vi "getPointFromEnemyOrientationAndBallToOurGoal.vi"(8 "error in (no error)":errorcluster, 9 "Robot":refnum<class "Robot.lvclass">, 10 "Game":refnum<class "Game.lvclass">, 11 "Utilities in":refnum<class "Utilities.lvclass">) -> (0 "error out":errorcluster, 1 "y_intersection":dbl, 2 "x_intersection":dbl, 3 "Utilities out":refnum<class "Utilities.lvclass">)   [LabVIEW 2018, in "Utilities.lvclass"]
uses:
  Utilities.lvclass
  Game_class/Game.lvclass
  Robot_class/Robot.lvclass
  Game_class/Game.lvclass/Game.ctl
  Robot_class/Robot.lvclass/Robot.ctl
  Object_class/Object.lvclass/Object.ctl
  Robot_class/Read orientation.vi
  Game_class/Read FieldRef.vi
  Game_class/Read BallRef.vi
  Object_class/Read x.vi
  Object_class/Read y.vi
  Ball_class/Ball.lvclass
  C:/Users/Gustavo/Desktop/RoboIME/SimplePass/SSL_AI/Object_class/Object.lvclass
  Field_class/Field.lvclass
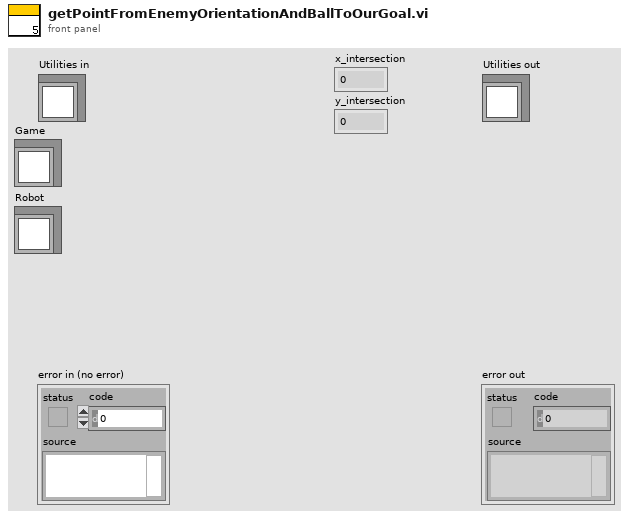
[diagram p1: front panel]
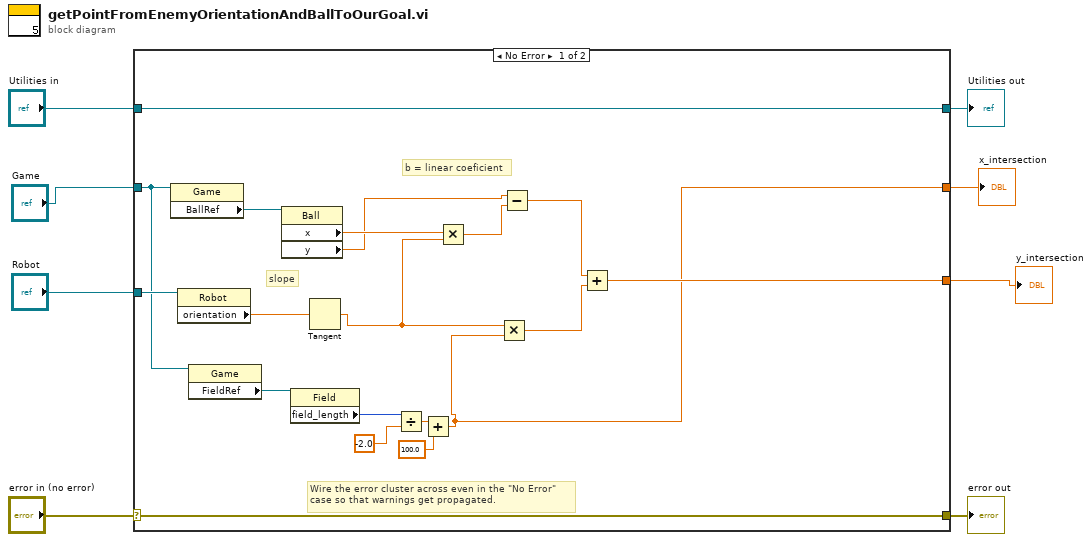
[diagram p0: block diagram]
diagram:
  n1 = case shown="No Error" "error in (no error)" {
    selector: "error in (no error)" -> [w26 w29]
    tunnel: [w26 w29] -> w7
    tunnel: [w27 w28] -> w5
    tunnel: "Utilities in" -> [w27 w28]
    tunnel: "Game" -> [w22 _]
    tunnel: "Robot" -> [w24 _]
    tunnel: [w11 _] -> w2
    tunnel: [w12 _] -> w1
    frame No Error {
      # "slope"
      # "b = linear coeficient"
      # "Wire the error cluster across even in the \"No Error\"\ncase so that warnings get propagated."
      n2 = property class="Game"(reference=w22) -> ("BallRef"=w25:refnum<class "Ball.lvclass">)  [unwired: 1 in, 2 out]
      n3 = property class="Robot"(reference=w24) -> ("orientation"=w23:dbl)  [unwired: 1 in, 2 out]
      n4 = property class="Game"(reference=w22) -> ("FieldRef"=w21:refnum<class "Field.lvclass">)  [unwired: 1 in, 2 out]
      n5 = property class="Ball"(reference=w25) -> ("x"=w18:dbl, "y"=w16:dbl)  [unwired: 1 in, 2 out]
      n6 = property class="Field"(reference=w21) -> ("field_length"=w20:i32)  [unwired: 1 in, 2 out]
      n7 = Tangent(1:w23) -> (0:w17:dbl)
      n8 = Divide(x=w20, y=-2.0) -> (x/y=w10:dbl)
      n9 = Add(x=w10, y=100.0) -> (x+y=w11:dbl)
      n10 = Multiply(x=w18, y=w17) -> (x*y=w15:dbl)
      n11 = Multiply(x=w17, y=w11) -> (x*y=w14:dbl)
      n12 = Subtract(x=w16, y=w15) -> (x-y=w13:dbl)
      n13 = Add(x=w13, y=w14) -> (x+y=w12:dbl)
    }
    frame Error {
    }
  }
  "error out" <- w7
  "Utilities out" <- w5
  "x_intersection" <- w2
  "y_intersection" <- w1
